vi "test Set Variant.vi"(8 "error in (no error)":errorcluster, 11 "TestCase in":refnum<class "UUID Structure Tests.lvclass">) -> (0 "error out":errorcluster, 3 "TestCase out":refnum<class "UUID Structure Tests.lvclass">)   [LabVIEW 2015, in "UUID Structure Tests.lvclass"]
uses:
  UUID Structure Tests.lvclass
  UUID/Variants.ctl
  <vilib>/addons/_JKI Toolkits/VI Tester/TestCase.llb/TestCase.lvclass
  UUID/UUID.lvclass
  <vilib>/Wiresmith Technology/VITAC (VI Tester Advanced Comparisons)/VITAC.lvlib
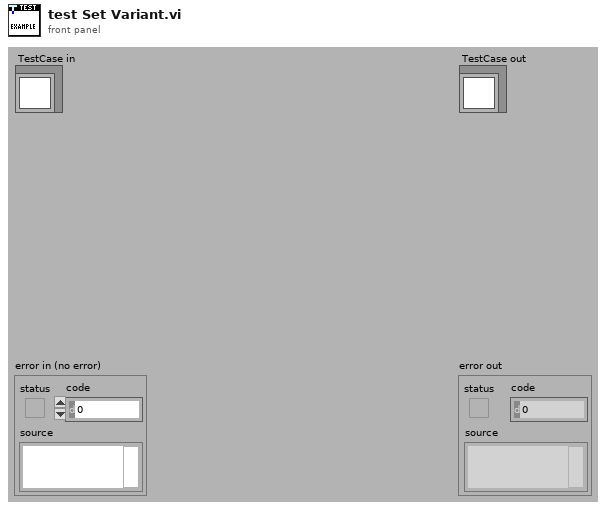
[diagram p1: front panel]
types:
  T1 = typedef "UUID.lvclass/Variants.ctl" = enum16{"NCS", "RFC", "Microsoft"}
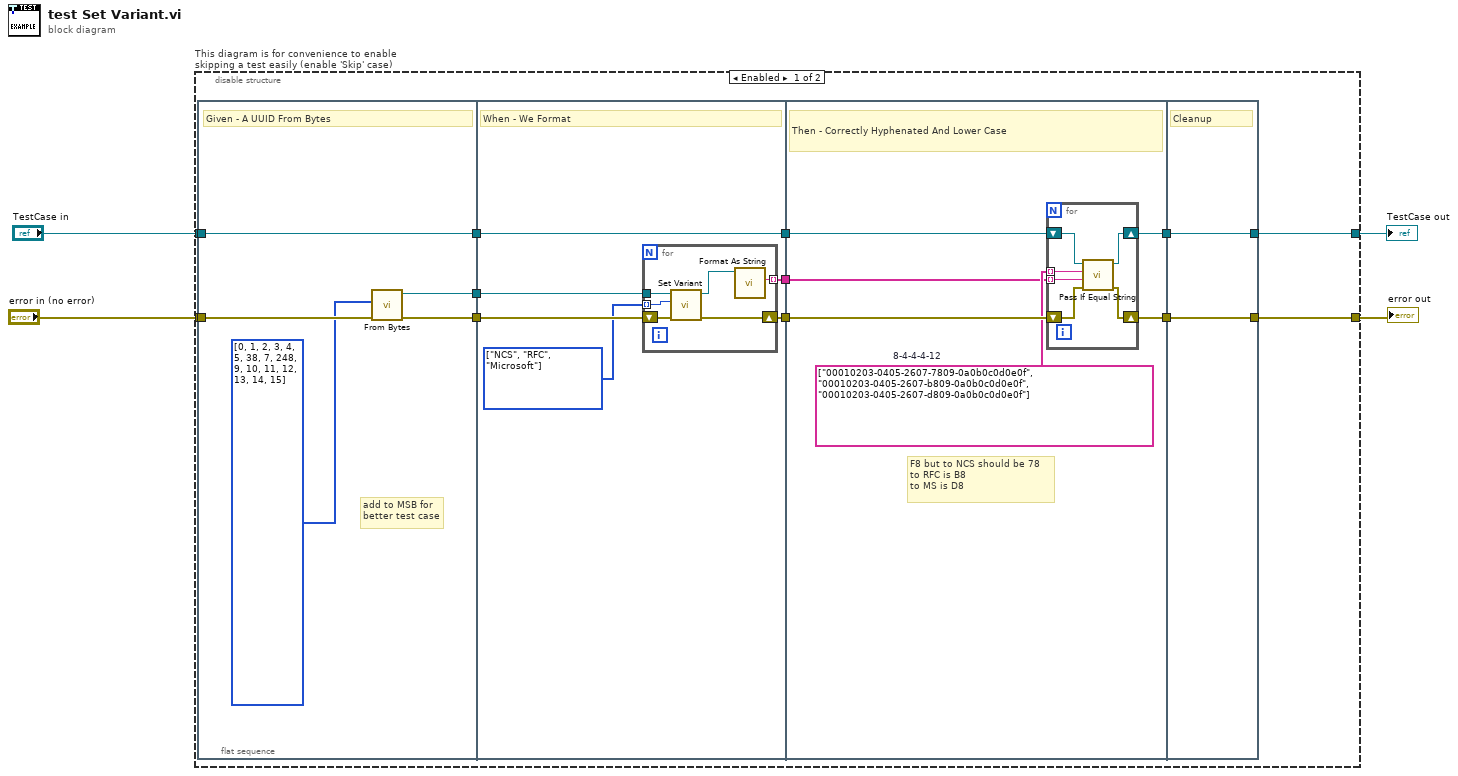
[diagram p0: block diagram]
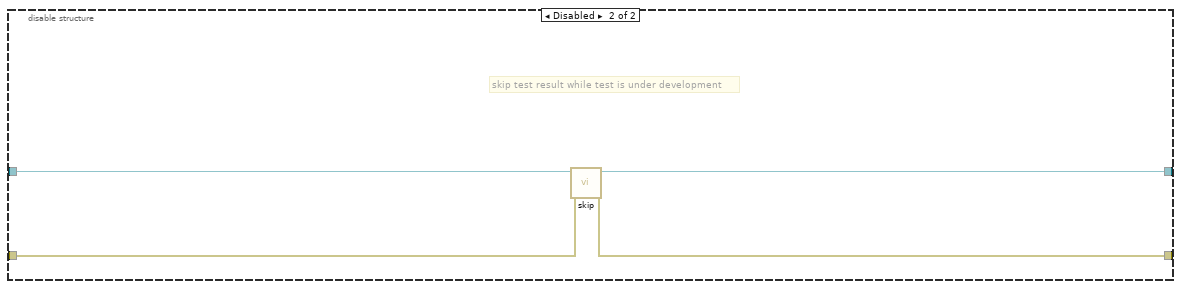
[diagram p2: hidden frame]
diagram:
  n1 = disable-structure "This diagram is for convenience to enable skipping a test easily (enable 'Skip' case)" shown="Enabled" {
    disable-tunnel: "TestCase in" -> [w10 w51]
    disable-tunnel: [w8 w49] -> w1
    disable-tunnel: [w7 w50] -> w3
    disable-tunnel: "error in (no error)" -> [w9 w48]
    frame Enabled {
      n2 = flat-sequence {
        tunnel: w9 -> [w20]
        tunnel: w10 -> [w21]
        tunnel: [w21] -> w16
        tunnel: [w19] -> w15
        tunnel: [w18] -> w6
        tunnel: [w27] -> w14
        tunnel: [w25] -> w13
        tunnel: w16 -> [w27]
        tunnel: w15 -> [w26]
        tunnel: w6 -> [w24]
        tunnel: [w22] -> w5
        tunnel: [w38] -> w12
        tunnel: [w36] -> w11
        tunnel: w14 -> [w39]
        tunnel: w13 -> [w37]
        tunnel: w5 -> [w34]
        tunnel: [w46] -> w7
        tunnel: [w47] -> w8
        tunnel: w12 -> [w47]
        tunnel: w11 -> [w46]
        frame #0 {
          # "add to MSB for\nbetter test case"
          # "Given - A UUID From Bytes"
          n3 = call "From Bytes.vi"("error in (no error)"=w20, "Bytes"=u8[] [0, 1, 2, 3, 4, 5, 38, 7, 248, 9, 10, 11, 12, 13, 14, 15]) -> ("error out"=w19:errorcluster, "UUID out"=w18:refnum<class "UUID.lvclass">)  [unwired: 8 in]
        }
        frame #1 {
          w23 = T1[] [enum."NCS", enum."RFC", enum."Microsoft"] items=["NCS", "RFC", "Microsoft"] ("Variant")
          # "When - We Format"
          n4 = for {
            tunnel: w24 -> [w31]
            tunnel: w23 -> [w30] mode=indexing
            tunnel: [w28] -> w22 mode=indexing
            shift-right: [w32] -> w25
            shift-left: w26 -> [w33]
            n5 = call "Set Variant.vi"("error in (no error)"=w33, "Variant (RFC)"=w30, "UUID in"=w31) -> ("error out"=w32:errorcluster, "UUID out"=w29:refnum<class "UUID.lvclass">)  [unwired: 7 in]
            n6 = call "Format As String.vi"("UUID.lvclass"=w29) -> ("String"=w28:string)  [unwired: 10 in]
          }
        }
        frame #2 {
          w35 = string[] ["00010203-0405-2607-7809-0a0b0c0d0e0f", "00010203-0405-2607-b809-0a0b0c0d0e0f", "00010203-0405-2607-d809-0a0b0c0d0e0f"]  # 8-4-4-4-12
          # "F8 but to NCS should be 78\nto RFC is B8\nto MS is D8"
          # "Then - Correctly Hyphenated And Lower Case"
          n7 = for {
            tunnel: w35 -> [w41] mode=indexing
            tunnel: w34 -> [w40] mode=indexing
            shift-right: [w44] -> w38
            shift-left: w39 -> [w45]
            shift-right: [w42] -> w36
            shift-left: w37 -> [w43]
            n8 = call <vilib>:"Pass If Equal String.vi"("error in (no error)"=w43, "actual"=w40, "expected"=w41, "TestCase in"=w45) -> ("error out"=w42:errorcluster, "TestCase out"=w44:refnum<class "UUID Structure Tests.lvclass">)  [unwired: 6 in]
          }
        }
        frame #3 {
          # "Cleanup"
        }
      }
    }
    frame Disabled {
      # "skip test result while test is under development"
      n9 = call <vilib>:"skip.vi"("error in (no error)"=w48, "TestCase in"=w51) -> ("error out"=w50:errorcluster, "TestCase out"=w49:refnum<class "UUID Structure Tests.lvclass">)  [unwired: 8 in]
    }
  }
  "error out" <- w3
  "TestCase out" <- w1
